vi "Broadcast.vi"(8 "error in (no error)":errorcluster, 9 "Data":string, 10 "ID":string, 11 "Websocket Server in":refnum<class "Websocket Server.lvclass">) -> (0 "error out":errorcluster, 3 "Websocket Server out":refnum<class "Websocket Server.lvclass">)   [LabVIEW 2020]
uses:
  Websocket Server.lvclass/Websocket Server.ctl
  Websocket Server.lvclass
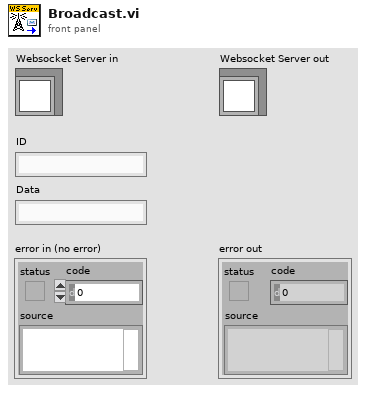
[diagram p1: front panel]
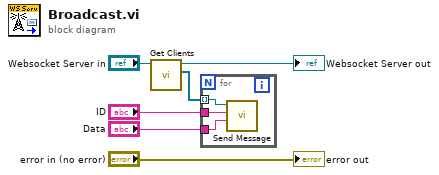
[diagram p0: block diagram]
diagram:
  n1 = call "Get Clients.vi"("Websocket Server in"="Websocket Server in") -> ("Clients"=w4:refnum<class "Websocket Client.lvclass">[], "Websocket Server out"=→"Websocket Server out":refnum<class "Websocket Server.lvclass">)  [unwired: 8 in, 1 out]
  n2 = for {
    tunnel: w4 -> [w9] mode=indexing
    tunnel: "ID" -> [w8]
    tunnel: "Data" -> [w7]
    n3 = call "Send Message.vi"("Data"=w7, "ID"=w8, "Websocket Client in"=w9) -> ()  [unwired: 7 in, 2 out]
  }
  "error out" <- "error in (no error)"
